vi "ArraySize.vi"() -> ()   [LabVIEW 2019]
panel:
  out "size(s) 2":i32[](array[numeric])
  in  "a 2D":u8[][](array[numeric])=[[10, 20, 30, 40, 50]]
  out "size(s)":i32
  in  "a":u8[](array[numeric])=[10, 20, 30, 40, 50]
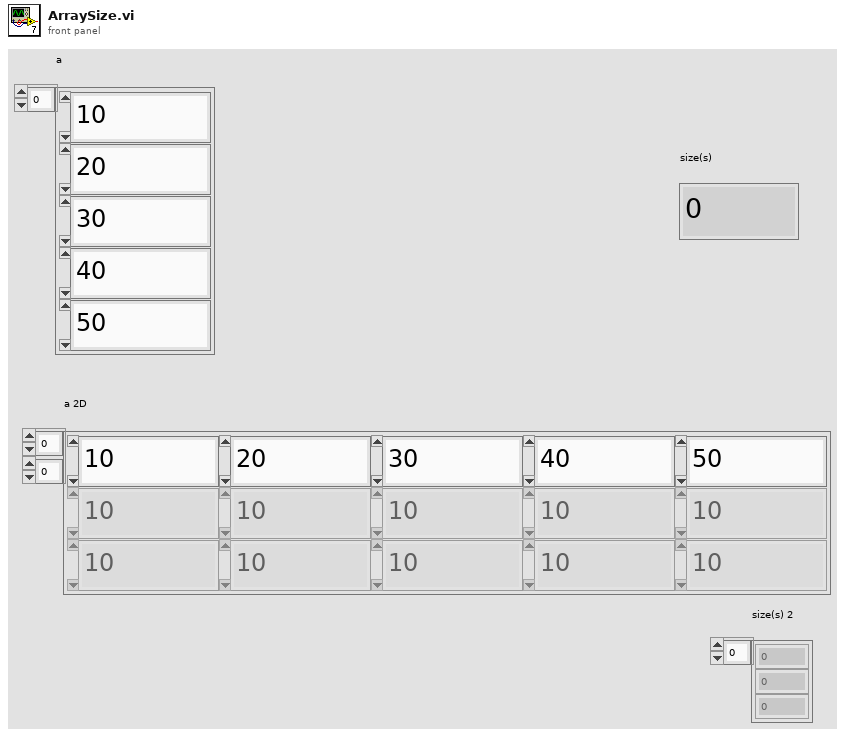
[diagram p1: front panel]
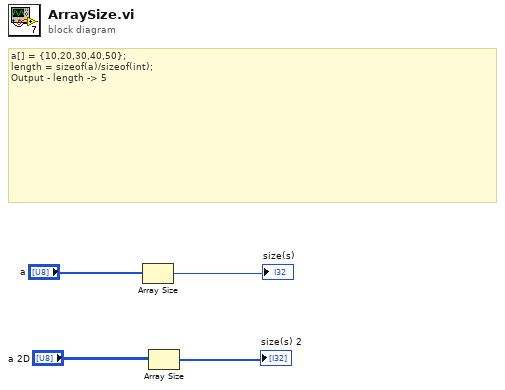
[diagram p0: block diagram]
diagram:
  # "a[] = {10,20,30,40,50};\nlength = sizeof(a)/sizeof(int);\nOutput - length -> 5"
  n1 = Array Size(array="a") -> (size(s)=→"size(s)":i32)
  n2 = Array Size(array="a 2D") -> (size(s)=→"size(s) 2":i32[])
